vi "test No Configuration.vi"(8 "error in":errorcluster, 11 "reference in":refnum<class "AIM ARINC 664 Deployment.lvclass">) -> (0 "error out":errorcluster, 3 "reference out":refnum<class "AIM ARINC 664 Deployment.lvclass">)   [LabVIEW 2020, in "AIM ARINC 664 Deployment.lvclass"]
uses:
  AIM ARINC 664 Deployment.lvclass
  AIM ARINC 664 Deployment.lvclass/AIM ARINC 664 Deployment.ctl
  b396e5f9-bef9-40c7-8d06-c3a1c8b08d2b.vi
  4719baa5-4bfd-4fe5-bb7f-2dd118eb5335.vi
  <vilib>/addons/_JKI Toolkits/VI Tester/TestCase.llb/TestCase.lvclass
  C:/Program Files (x86)/National Instruments/LabVIEW 2020/vi.lib/NI/VeriStand Custom Device Testing Tools/VeriStandTestCase/VeriStandTestCase.lvclass
  C:/Program Files (x86)/National Instruments/LabVIEW 2020/vi.lib/addons/_JKI Toolkits/VI Tester/TestCase.llb/TestCase.lvclass
  C:/Users/Administrator/Desktop/git/niveristand-aim-arinc664-custom-device/Source/Custom Device Support/Tests/System/AIM_Deployment/AIM ARINC 664 Deployment.lvclass
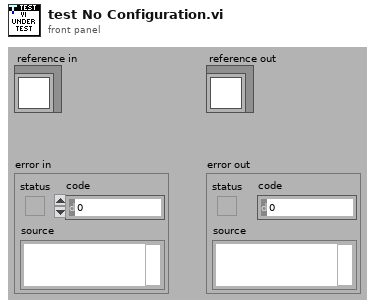
[diagram p1: front panel]
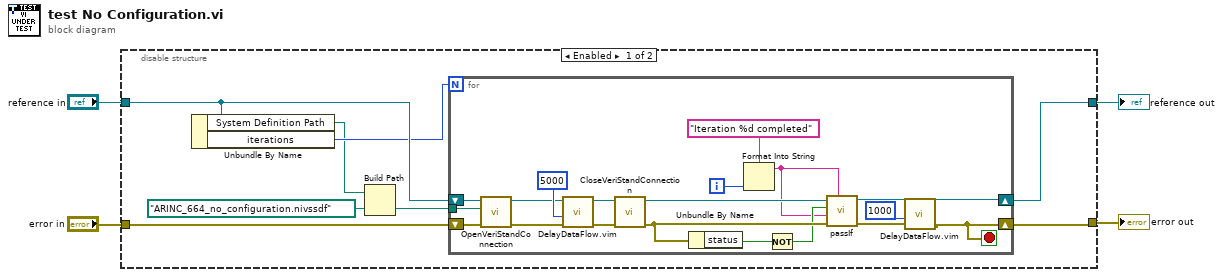
[diagram p0: block diagram]
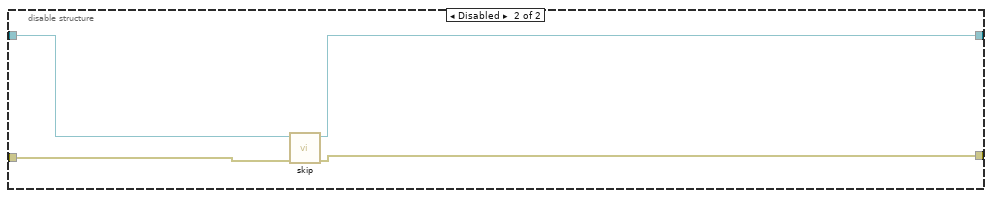
[diagram p2: hidden frame]
diagram:
  n1 = disable-structure shown="Enabled" {
    disable-tunnel: "reference in" -> [w12 w34]
    disable-tunnel: "error in" -> [w11 w33]
    disable-tunnel: [w10 w32] -> w2
    disable-tunnel: [w9 w31] -> w1
    frame Enabled {
      n2 = Unbundle By Name(w12) -> ("System Definition Path"=w6:path, "iterations"=w8:i32)
      n3 = Build Path(base path=w6, name or relative path=path "ARINC_664_no_configuration.nivssdf") -> (appended path=w7:path)
      n4 = for {
        N: w8 -> [_]
        tunnel: w7 -> [w24]
        shift-right: [w19] -> w9
        shift-left: w12 -> [w28]
        shift-right: [w13] -> w10
        shift-left: w11 -> [w27]
        i -> [w18]
        stop <- w13 stop-if-true
        n5 = call-dynamic "OpenVeriStandConnection.vi"("error in (no error)"=w27, "System Definition File"=w24, "VeriStand Test Case in"=w28) -> ("error out"=w26:errorcluster, "VeriStand Test Case out"=w25:refnum<class "AIM ARINC 664 Deployment.lvclass">)  [unwired: 6 in, 1 out]
        n6 = call "DelayDataFlow.vim"("value in"=w26, "milliseconds to wait"=u32 5000) -> ("value out"=w30:errorcluster)  [unwired: 2 in, 1 out]
        n7 = call-dynamic "CloseVeriStandConnection.vi"("error in (no error)"=w30, "VeriStand Test Case in"=w25) -> ("error out"=w23:errorcluster, "VeriStand Test Case out"=w20:refnum<class "AIM ARINC 664 Deployment.lvclass">)  [unwired: 8 in]
        n8 = Unbundle By Name(w23) -> ("status"=w22:bool)
        n9 = Format Into String(format string="Iteration %d completed", w18) -> (resulting string=w16:string)  [unwired: 2 in, 1 out]
        n10 = Not(x=w22) -> (.not. x?=w21:bool)
        n11 = call-dynamic "passIf.vi"("custom report message (\"\")"=w16, "error in (no error)"=w23, "message (\"\")"=w16, "pass"=w21, "TestCase in"=w20) -> ("error out"=w14:errorcluster, "TestCase out"=w19:refnum<class "AIM ARINC 664 Deployment.lvclass">)  [unwired: 5 in]
        n12 = call "DelayDataFlow.vim"("value in"=w14, "milliseconds to wait"=u32 1000) -> ("value out"=w13:errorcluster)  [unwired: 2 in, 1 out]
      }
    }
    frame Disabled {
      n13 = call <vilib>:"skip.vi"("error in (no error)"=w33, "TestCase in"=w34) -> ("error out"=w32:errorcluster, "TestCase out"=w31:refnum<class "AIM ARINC 664 Deployment.lvclass">)  [unwired: 8 in]
    }
  }
  "error out" <- w2
  "reference out" <- w1
